vi "Check for duplicate channels.vi"() -> ()   [LabVIEW 2022 SP3]
uses:
  Sub VIs/ADAM Controls/Channel_names.ctl
  Sub VIs/ADAM Controls/Address.ctl
  Sub VIs/ADAM Controls/Module_type_ADAM.ctl
  Sub VIs/ADAM Controls/Function_ADAM.ctl
  Sub VIs/ADAM Controls/Channel_State.ctl
  Sub VIs/ADAM Controls/Calib_type_ADAM.ctl
  Sub VIs/ADAM Controls/Ch_description_ADAM.ctl
panel:
  out "Array":T7(array[cluster]) {"Ch Discription"."Duty" format="%016b"; "Ch Discription"."D" format="%#_5g"; "Ch Discription"."C" format="%#_5g"; "Ch Discription"."B" format="%#_5g"; "Ch Discription"."A" format="%#_5g"; "Ch Discription"."Duty" format="%016b"; "Ch Discription"."D" format="%#_5g"; "Ch Discription"."C" format="%#_5g"; "Ch Discription"."B" format="%#_5g"; "Ch Discription"."A" format="%#_5g"}
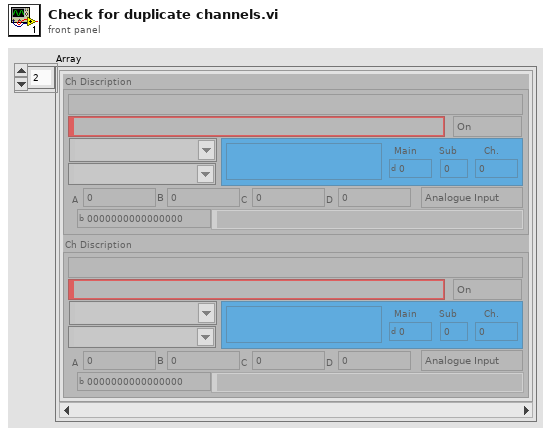
[diagram p1: front panel]
types:
  T1 = typedef "Ch_description_ADAM.ctl" = cluster{"Ch Name":string, "Type":T2, "Function":T3, "Ch State":T4, "Calibration type":T5, "A":dbl, "B":dbl, "C":dbl, "D":dbl, "Comments":string, "Address":T6, "String":string, "Duty":u16}
  T2 = typedef "Module_type_ADAM.ctl" = string
  T3 = typedef "Function_ADAM.ctl" = enum16{"Analogue Input", "Digital Input", "Event counter", "Event rate", "Analogue Output", "Digital Output", "Relay Output"}
  T4 = typedef "Channel_State.ctl" = enum16{"On", "Off", "Always On", "Always Off"}
  T5 = typedef "Calib_type_ADAM.ctl" = string
  T6 = typedef "Address.ctl" = cluster{"Main":i32, "Ch.":i32, "Sub":i32, "Port Name":string}
  T7 = cluster{"Ch Discription":T1, "Ch Discription":T1}[]
  T8 = typedef "Channel_names.ctl" = enum16{"Active Only", "Active + Off", "All Channels", "Changeable Only"}
  T9 = cluster{"Ch Discription":T1, "Ch Discription":T1}
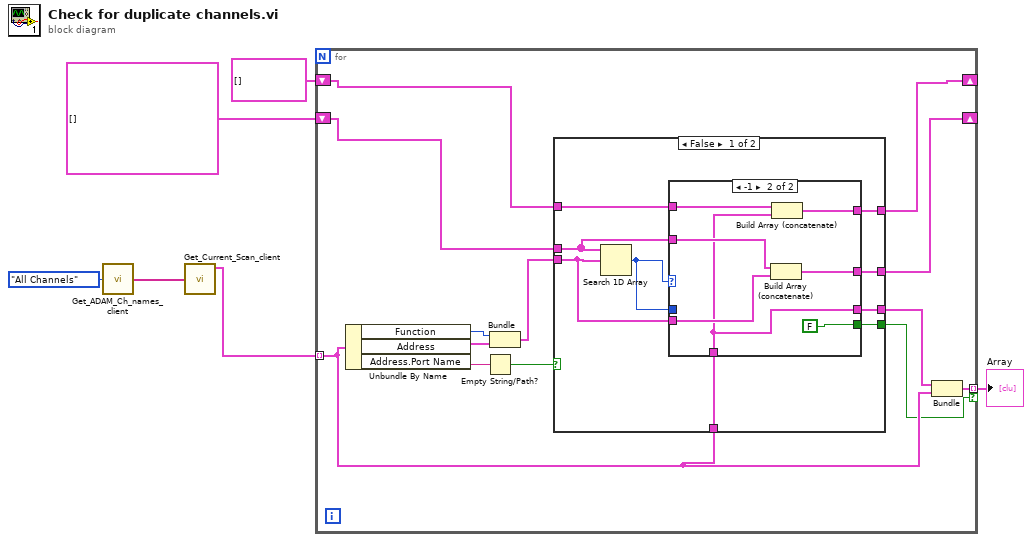
[diagram p0: block diagram]
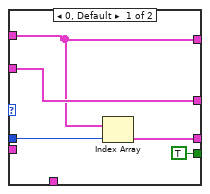
[diagram p2: hidden frame]
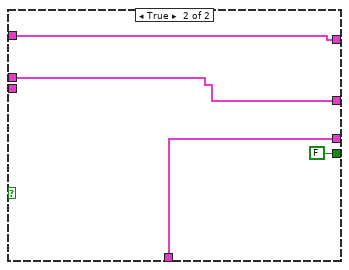
[diagram p3: hidden frame]
diagram:
  n1 = call "Get_ADAM_Ch_names_client.vi"("Channel names set"=Channel_names."All Channels") -> ("Ch names"=w5:string[])
  n2 = call "Get_Current_Scan_client.vi"("ADAM Ch Names"=w5) -> ("Ch Description Array"=w4:T1[])  [unwired: 3 out]
  n3 = for {
    tunnel: w4 -> [w12] mode=indexing
    shift-right: [w16] -> _
    shift-left: cluster{"Function":T3, "Address":T6}[] [] -> [w17]
    shift-right: [w15] -> _
    shift-left: T1[] [] -> [w14]
    tunnel: [w11] -> w2 mode=indexing if=w10
    n4 = Unbundle By Name(w12) -> ("Function"=w8:T3, "Address"=w9:T6, "Address.Port Name"=w19:string)
    n5 = Empty String/Path?(string/path=w19) -> (empty?=w18:bool)
    n6 = Bundle("Function"=w8, "Address"=w9) -> (w7:cluster{"Function":T3, "Address":T6})  [unwired: 1 in]
    n7 = case shown="False" w18 {
      tunnel: w17 -> [w28 w43]
      tunnel: w7 -> [w27 _]
      tunnel: [w26 w43] -> w16
      tunnel: [w25 FALSE] -> w10
      tunnel: [w24 w41] -> w15
      tunnel: w14 -> [w23 w41]
      tunnel: w12 -> [w22 w42]
      tunnel: [w20 w42] -> w13
      frame False {
        n8 = Search 1D Array(1D array=w28, element=w27) -> (index of element=w21:i32)  [unwired: 1 in]
        n9 = case shown="-1" w21 {
          tunnel: w28 -> [w33 w40]
          tunnel: w27 -> [_ w39]
          tunnel: [w33 w38] -> w26
          tunnel: [TRUE FALSE] -> w25
          tunnel: [w30 w36] -> w24
          tunnel: w23 -> [w30 w35]
          tunnel: w22 -> [_ w34]
          tunnel: w21 -> [w31 _]
          tunnel: [w29 w34] -> w20
          frame 0, Default {
            n10 = Index Array(array=w30, index=w31) -> (element=w29:T1)
          }
          frame -1 {
            n11 = Build Array (concatenate)(w40, w39) -> (w38:cluster{"Function":T3, "Address":T6}[])
            n12 = Build Array (concatenate)(w35, w34) -> (w36:T1[])
          }
        }
      }
      frame True {
      }
    }
    n13 = Bundle("Ch Discription"=w13, "Ch Discription"=w12) -> (w11:T9)  [unwired: 1 in]
  }
  "Array" <- w2
